vi "MessageEditor.vi"() -> ()   [LabVIEW 2019]
uses:
  simonMessages.lvclass
panel:
  in  "Messages Table":string[][](table)=[["welcome", "Welcome\r\nto\r\nLabVIEW Simon\r\nby\r\nFelipe Flores\r\n", "25", "Center", "LineByLine"], ["instructions", "\n\nSlide \"LEVEL\" to see how good you are.\n\nPress \"PLAY\" to start playing.\n\nPress \"LONGEST\" to see the longest sequence ever played.", "16", "Center", "Plain"], ["stageUp", "\\n\\rStage\\s%d", "60", "Center", "Rotate"], ["startGame", "\nLet's do it!", "40", "Center", "Plain"], ["last", "\nPlaying last Sequence...", "40", "Left", "Plain"], ["longest", "\nPlaying longest Sequence...", "40", "Left", "Plain"], ["hsHeaders", "High,Scores\r\n=========,=========\r\n", "25", "Center", "LineByLine"], ["levelChoice", "Level %d selected", "", "Left", "Plain"], ["yourTurn", "\n\nyour turn!", "40", "Center", "Plain"], ["gameTitle", "Simon Game", "10", "Left", "TitleBar"], ["playerName", "%s is playing now!", "10", "Left", "TitleBar"]]
  in  "Filename":string
  in  "Save Button":bool
  in  "Open Button":bool
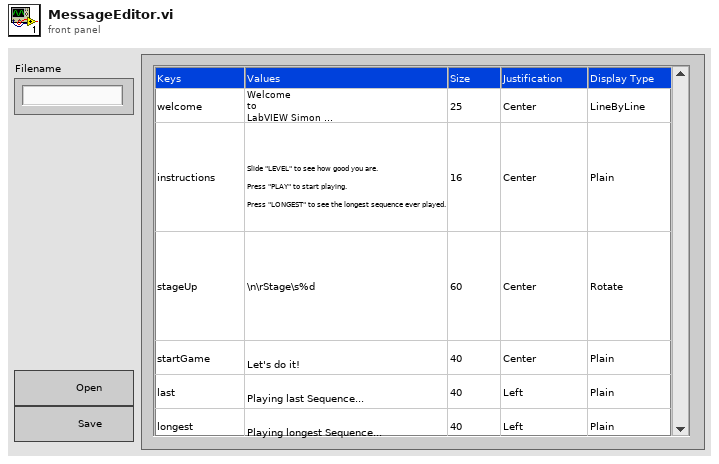
[diagram p1: front panel]
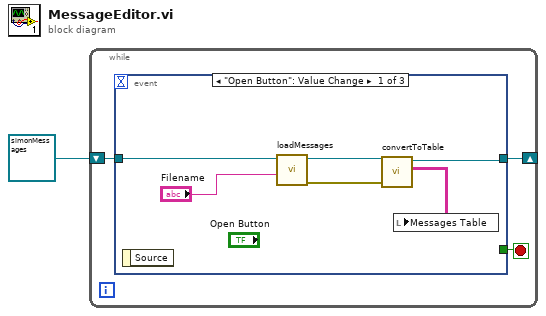
[diagram p0: block diagram]
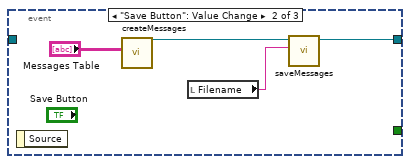
[diagram p2: hidden frame]
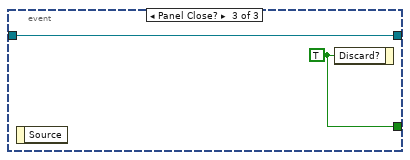
[diagram p3: hidden frame]
diagram:
  n1 = while {
    shift-right: [w3] -> _
    shift-left: refnum<class "simonMessages.lvclass"> refnum ("simonMessages.lvclass") -> [w4]
    stop <- w2 stop-if-true
    n2 = event shown="[0] \"Open Button\": Value Change" {
      selector: _ -> [_ _ _]
      dyn-events: _ -> [_ _ _]
      timeout: _ -> [_ _ _]
      tunnel: w4 -> [w10 _ w16]
      tunnel: [w7 w13 w16] -> w3
      tunnel: [_ _ w15] -> w2
      event "Open Button": Value Change {
        n3 = event-data() -> ()  [unwired: 1 in, 1 out]
        n4 = call "loadMessages.vi"("FileName (without extension)"="Filename", "simonMessages in"=w10) -> ("error out"=w6:errorcluster, "simonMessages out"=w8:refnum<class "simonMessages.lvclass">)  [unwired: 8 in]
        n5 = call "convertToTable.vi"("error in (no error)"=w6, "simonMessages in"=w8) -> ("Message table"=w5:string[][], "simonMessages out"=w7:refnum<class "simonMessages.lvclass">)  [unwired: 7 in, 1 out]
        n6 = local write "Messages Table"(w5) -> ()
      }
      event "Save Button": Value Change {
        n7 = event-data() -> ()  [unwired: 1 in, 1 out]
        n8 = call "createMessages.vi"("Messages Table"="Messages Table") -> ("simonMessages out"=w14:refnum<class "simonMessages.lvclass">)  [unwired: 9 in, 1 out]
        n9 = local read "Filename"() -> (w12:string)
        n10 = call "saveMessages.vi"("FileName (without extension)"=w12, "simonMessages in"=w14) -> ("simonMessages out"=w13:refnum<class "simonMessages.lvclass">)  [unwired: 8 in, 1 out]
      }
      event Panel Close? {
        w15 = TRUE ("Discard?")
        n11 = event-data() -> ()  [unwired: 1 in, 1 out]
        n12 = event-data("Discard?"=w15) -> ()  [unwired: 1 in, 1 out]
      }
    }
  }
